vi "Twos Complement.vi"(1 "Number":i16 format="%b") -> (0 "As Two's Complement":i16)   [LabVIEW 2015]
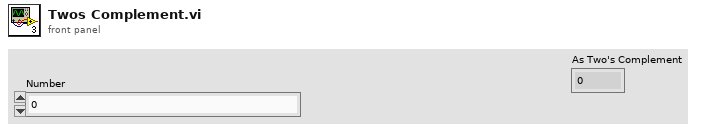
[diagram p1: front panel]
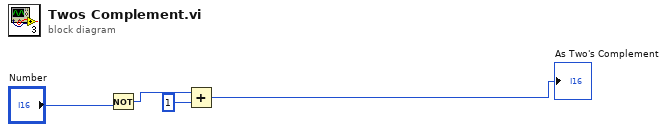
[diagram p0: block diagram]
diagram:
  n1 = Not(x="Number") -> (.not. x?=w3:i16)
  n2 = Add(x=w3, y=i16 1) -> (x+y=→"As Two's Complement":i16)
